vi "HighSpeedDemo.vi"() -> ()   [LabVIEW 2015]
uses:
  <vilib>/Platform/NI_3dgraph.lvlib
panel:
  out "Intensity Graph":dbl[][](graph)
  in  "3D Surface":refnum<k7>(container)
  out "Array":dbl[][](array[numeric])
  in  "number of Spectra":i32
  in  "Spectrometer Index":i32
  out "Number of Spectrometers":i32
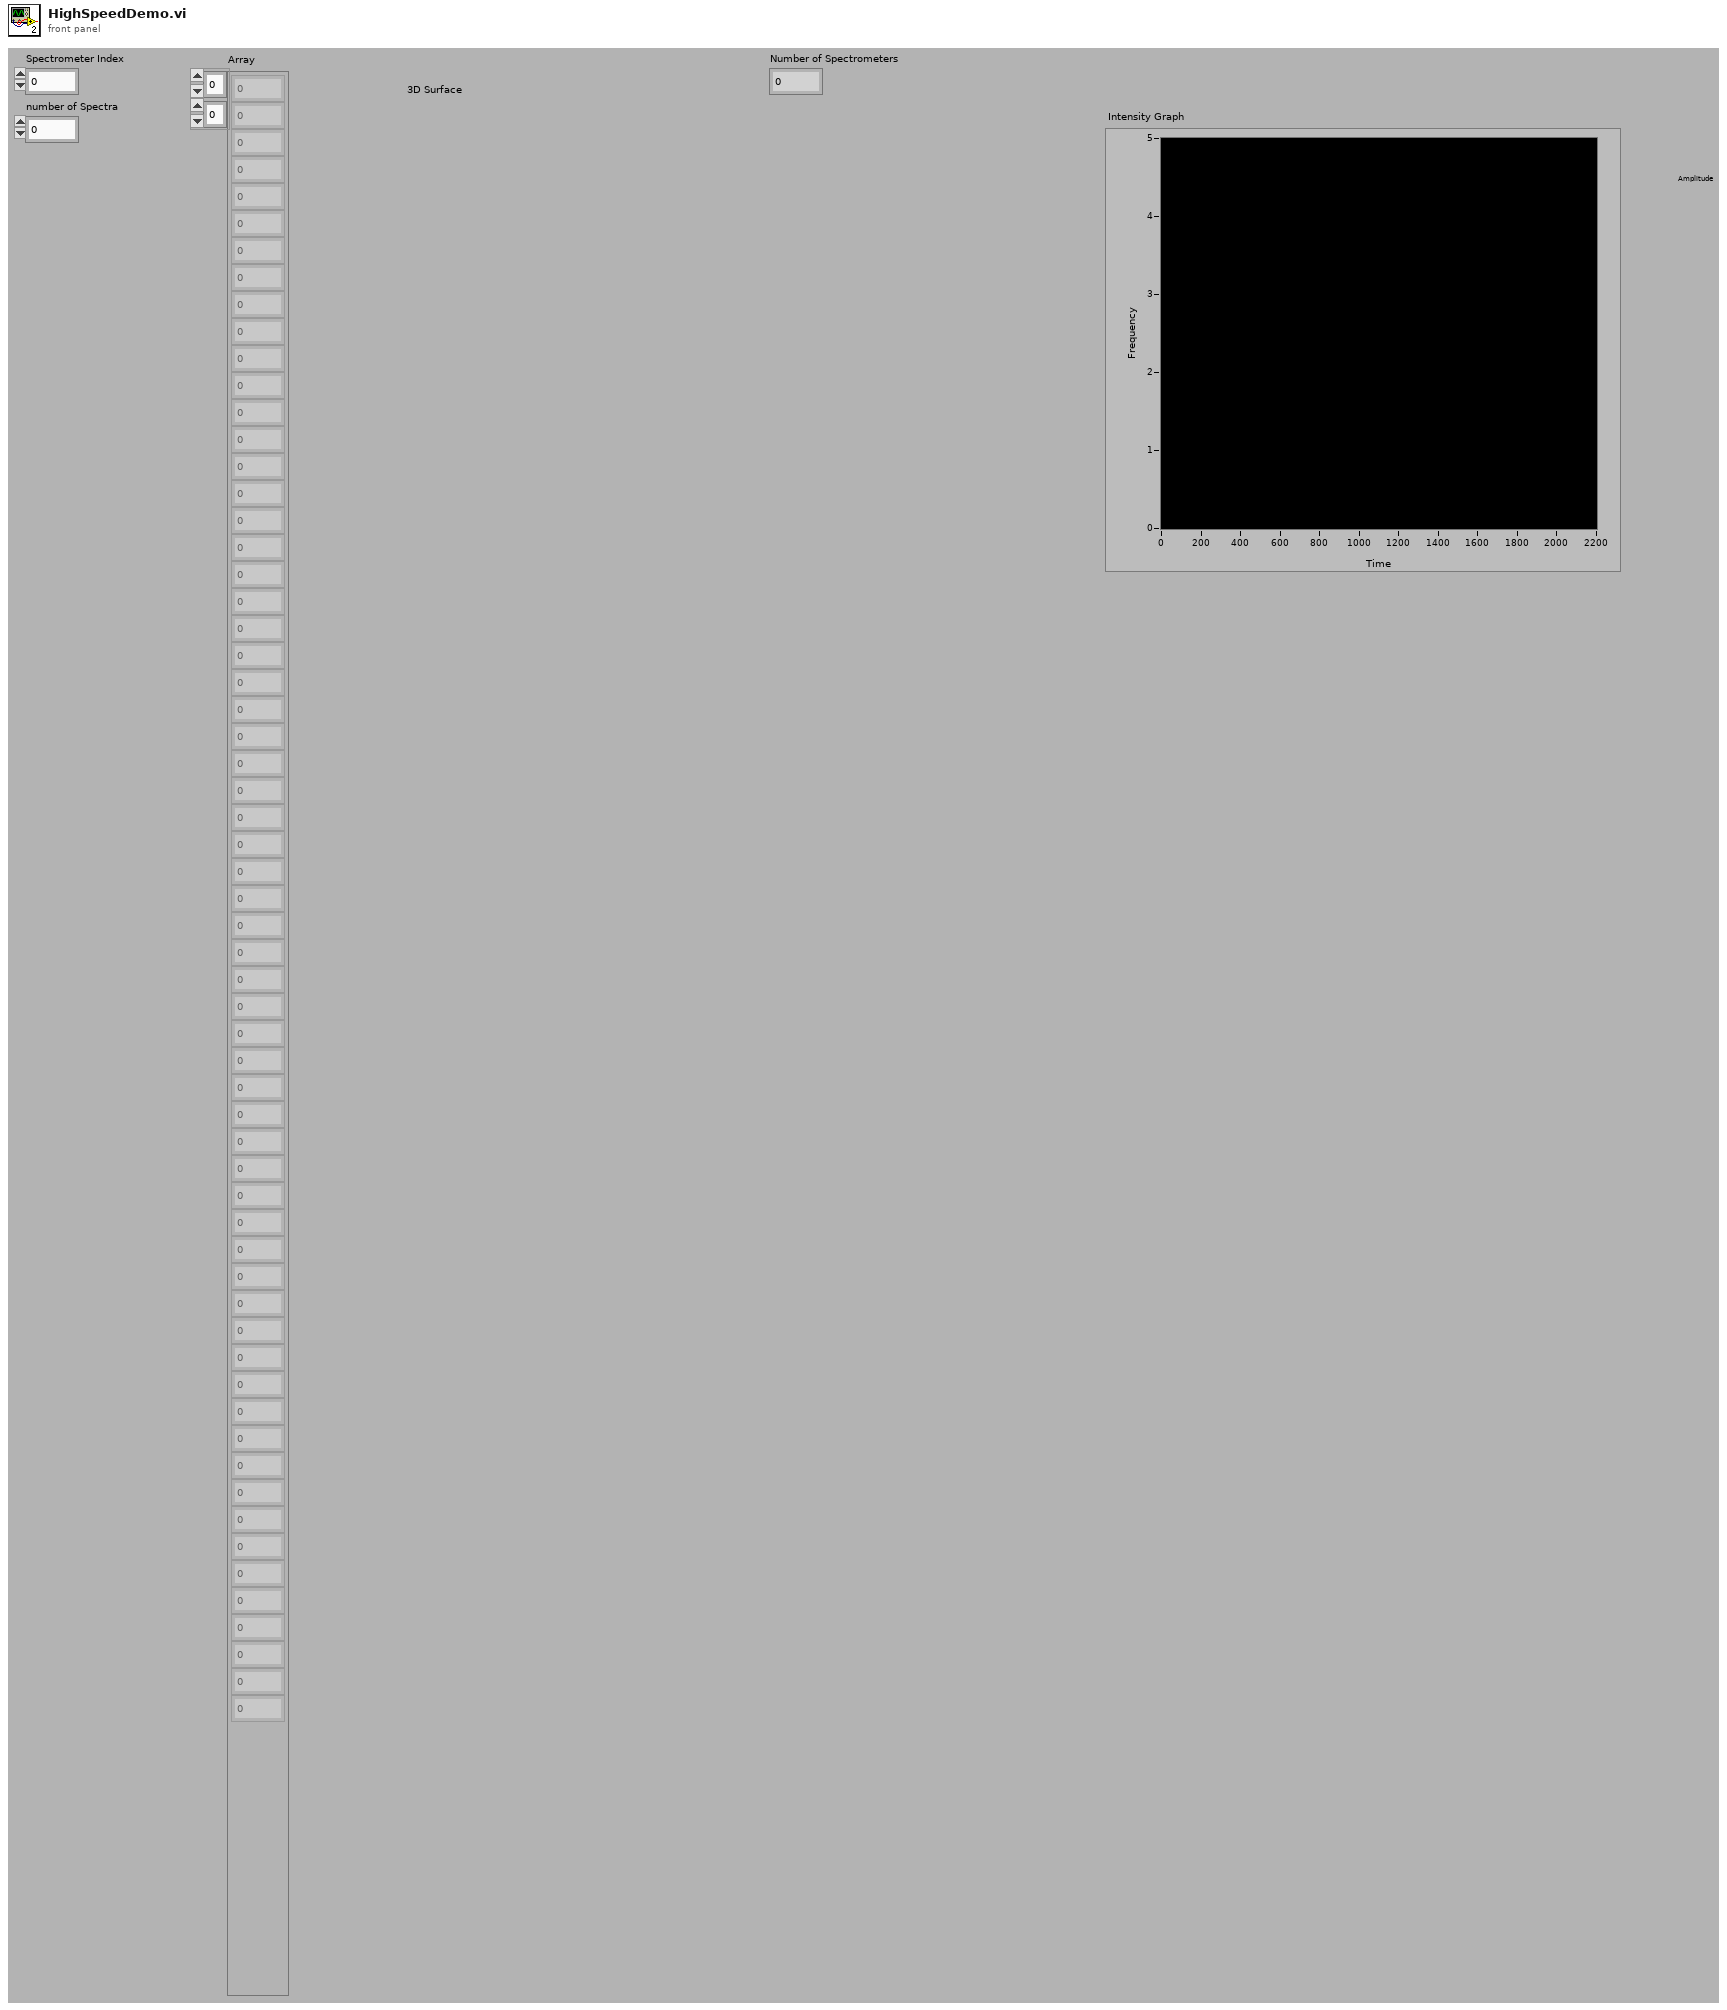
[diagram p1: front panel]
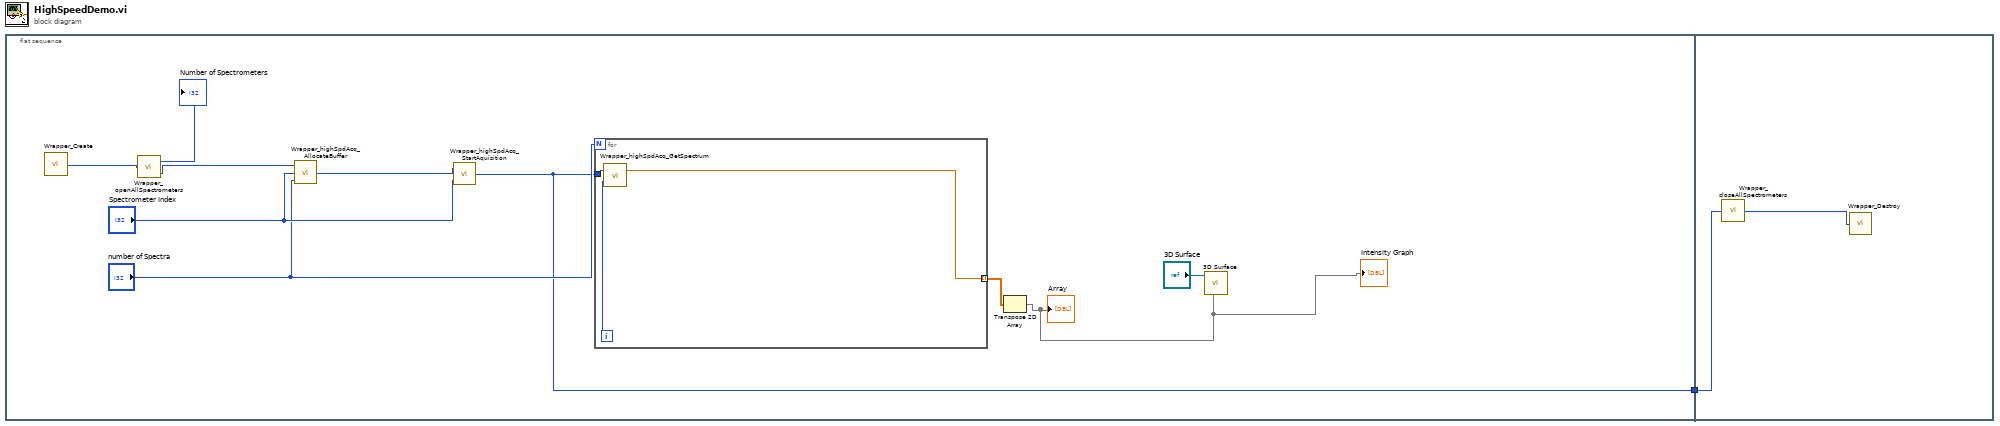
[diagram p0: block diagram]
diagram:
  n1 = flat-sequence {
    tunnel: [w5] -> w1
    tunnel: w1 -> [w15]
    frame #0 {
      n2 = call "Wrapper_Create.vi"() -> ("Wrapper"=w11:u32)
      n3 = call "Wrapper_openAllSpectrometers.vi"("Wrapper In"=w11) -> ("Number of Spectrometers"=→"Number of Spectrometers":i32, "Wrapper Out"=w10:u32)
      n4 = call "Wrapper_highSpdAcq_AllocateBuffer.vi"("number of Spectra"="number of Spectra", "Spectrometer Index"="Spectrometer Index", "Wrapper IN"=w10) -> ("Wrapper Out"=w8:u32)
      n5 = call "Wrapper_highSpdAcq_StartAquisition.vi"("Spectrometer Index"="Spectrometer Index", "Wrapper In"=w8) -> ("Wrapper Out"=w5:u32)
      n6 = for {
        N: "number of Spectra" -> [_]
        tunnel: w5 -> [w14]
        tunnel: [w12] -> w4 mode=indexing
        i -> [w13]
        n7 = call "Wrapper_highSpdAcq_GetSpectrum.vi"("Spectrum Number"=w13, "Wrapper"=w14) -> ("Spectrum Values"=w12:dbl[])  [unwired: 1 out]
      }
      n8 = Transpose 2D Array(2D array=w4) -> (transposed array=w2:dbl[][])
      "Array" <- w2
      "Intensity Graph" <- w2
      n9 = call <vilib>:"3D Surface.vi"("z matrix"=w2, "3D graph"="3D Surface") -> ()  [unwired: 8 in, 2 out]
    }
    frame #1 {
      n10 = call "Wrapper_closeAllSpectrometers.vi"("Wrapper In"=w15) -> ("Wrapper Out"=w16:u32)
      n11 = call "Wrapper_Destroy.vi"("Wrapper"=w16) -> ()
    }
  }
